vi "Download.vi"(7 "입력 클러스터":T1, 8 "에러 입력(에러 없음)":errorcluster, 10 "폴더명":path, 11 "TCP 네트워크 연결 입력":T2) -> (0 "에러 출력":errorcluster, 1 "다운로드 에러?":bool, 3 "TCP 네트워크 연결 출력":T2, 4 "타겟 경로":path, 5 "name":string, 6 "소스 경로":path)   [LabVIEW 2020]
uses:
  <vilib>/FTP/ftp0.llb/FTP Session.ctl
  <vilib>/Utility/sysdir.llb/System Directory Type.ctl
  <vilib>/security/Message Digest/API/Instances/File/SHA-256 File Checksum.vi
  <vilib>/security/Message Digest/API/NI_Message Digest API.lvlib
  <vilib>/FTP/NI_FTP.lvlib
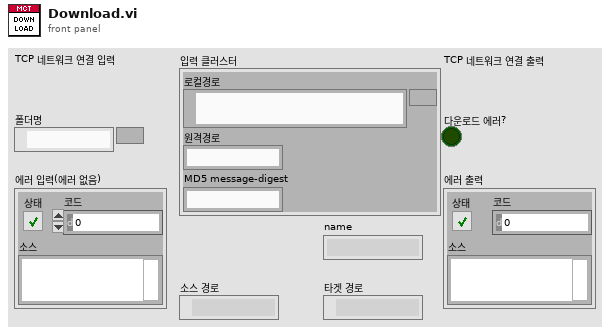
[diagram p1: front panel]
types:
  T1 = cluster{"로컬경로":path, "원격경로":string, "MD5 message-digest":string}
  T2 = typedef "NI_FTP.lvlib/FTP Session.ctl" = refnum<k5>
  T3 = typedef "System Directory Type.ctl" = i32
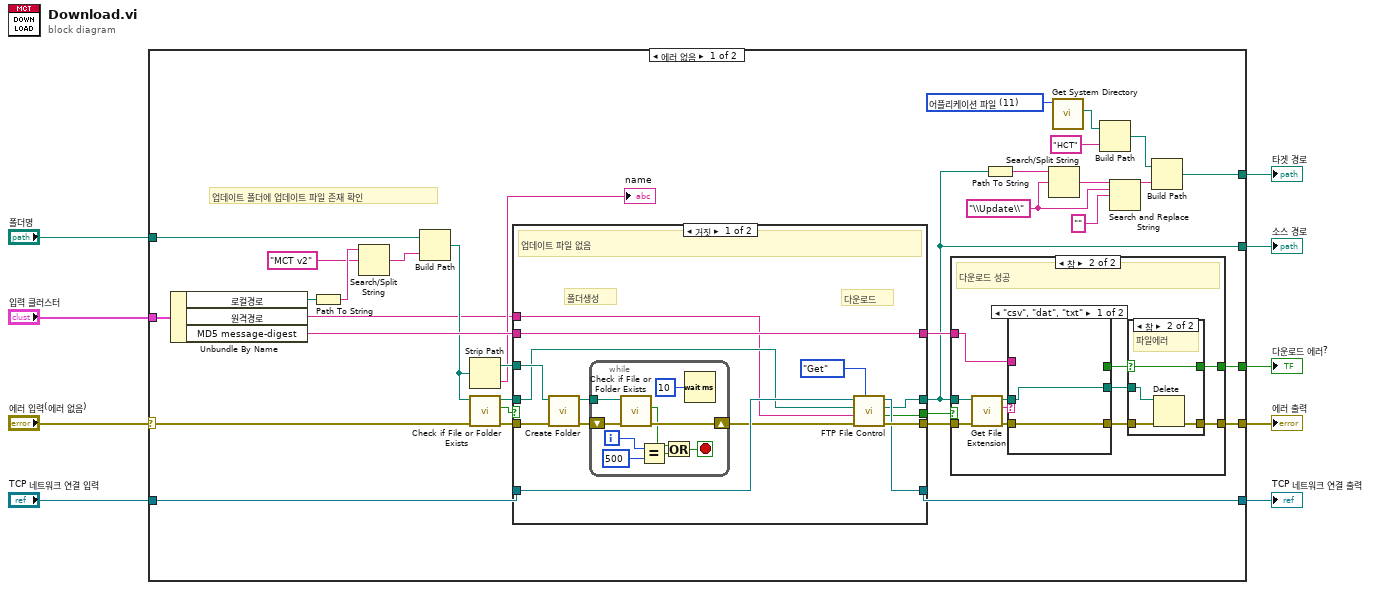
[diagram p0: block diagram]
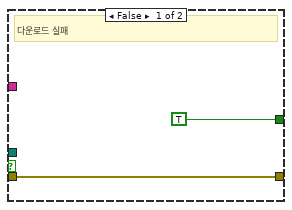
[diagram p2: hidden frame]
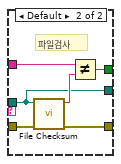
[diagram p3: hidden frame]
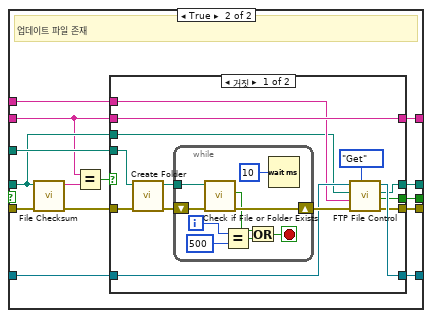
[diagram p5: hidden frame]
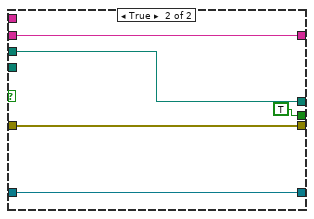
[diagram p6: hidden frame]
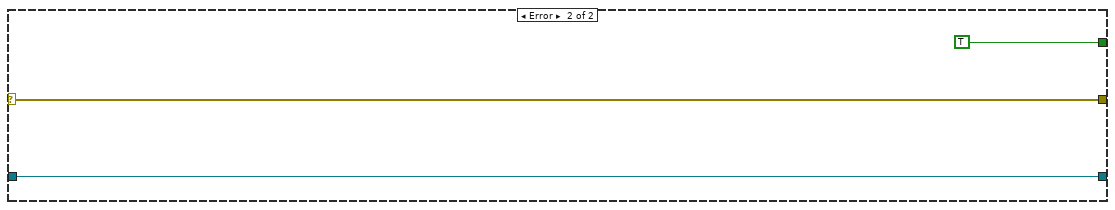
[diagram p7: hidden frame]
diagram:
  n1 = case shown="에러 없음" "에러 입력(에러 없음)" {
    selector: "에러 입력(에러 없음)" -> [w10 w135]
    tunnel: [w41 TRUE] -> w9
    tunnel: [w38 w135] -> w8
    tunnel: [w36 w137] -> w7
    tunnel: "TCP 네트워크 연결 입력" -> [w35 w137]
    tunnel: "폴더명" -> [w28 _]
    tunnel: "입력 클러스터" -> [w25 _]
    tunnel: [w21 _] -> w3
    tunnel: [w11 _] -> w2
    frame No Error {
      w16 = T3 11 items=["사용자 홈"=0, "사용자 데스크탑"=1, "사용자 문서"=2, "사용자 어플리케이션 데이터"=3, "사용자 환경"=4, "사용자 임시"=5, "퍼블릭 문서"=6, "퍼블릭 어플리케이션 데이터"=7, "퍼블릭 환경"=8, "퍼블릭 캐시"=13, "시스템 코어 라이브러리"=9, "시스템 설치된 라이브러리"=10, "어플리케이션 파일"=11, "부팅 볼륨 루트"=12] ("system directory type")
      w18 = "\\Update\\" ("검색 문자열/문자 (-)")
      # "업데이트 폴더에 업데이트 파일 존재 확인"
      n2 = Unbundle By Name(w25) -> ("로컬경로"=w24:path, "원격경로"=w23:string, "MD5 message-digest"=w40:string)
      n3 = Path To String(path=w24) -> (string=w27:string)
      n4 = Search/Split String(string=w27, search string/char (-)="MCT v2" ("검색 문자열/문자 (-)")) -> (match + rest of string=w29:string)  [unwired: 1 in, 2 out]
      n5 = Build Path(base path=w28, name or relative path=w29) -> (appended path=w39:path)
      n6 = Strip Path(path=w39) -> (stripped path=w34:path, name=→"name":string)
      n7 = call <vilib>:"Check if File or Folder Exists.vi"("error in (no error)"=w10, "path"=w39) -> ("error out"=w31:errorcluster, "file or folder exists?"=w32:bool, "dup path"=w33:path)  [unwired: 7 in]
      n8 = case shown="거짓" w32 {
        tunnel: w31 -> [w83 w106]
        tunnel: w33 -> [w71 w101]
        tunnel: w40 -> [w75 w94]
        tunnel: w34 -> [w79 w102]
        tunnel: w35 -> [w81 w100]
        tunnel: [w80 w99] -> w36
        tunnel: [w82 w98] -> w37
        tunnel: w23 -> [w70 w97]
        tunnel: [w73 w96] -> w21
        tunnel: [w74 w95] -> w42
        tunnel: [w75 w93] -> w22
        frame False {
          # "다운로드"
          # "폴더생성"
          # "업데이트 파일 없음"
          n9 = call "Create Folder.vi"("에러 입력"=w83, "폴더경로"=w79) -> ("error out"=w78:errorcluster, "dup path"=w77:path)  [unwired: 8 in]
          n10 = while {
            shift-right: [w91] -> w76
            shift-left: w78 -> [w92]
            tunnel: w77 -> [w90]
            i -> [w86]
            stop <- w88 stop-if-true
            n11 = call <vilib>:"Check if File or Folder Exists.vi"("error in (no error)"=w92, "path"=w90) -> ("error out"=w91:errorcluster, "file or folder exists?"=w89:bool)  [unwired: 7 in, 1 out]
            n12 = Equal?(x=w86, y=500) -> (x = y?=w87:bool)
            n13 = Or(x=w89, y=w87) -> (x .or. y?=w88:bool)
            n14 = Wait (ms)(milliseconds to wait=u32 10 ("대기 시간(ms)")) -> ()  [unwired: 1 out]
          }
          n15 = call "FTP File Control.vi"("Comm"=enum16{"Get", "Put"}."Get", "에러 입력"=w76, "원격경로"=w70, "로컬경로"=w71, "TCP 네트워크 연결 입력"=w81) -> ("에러 출력"=w82:errorcluster, "파일존재?"=w74:bool, "로컬경로 out"=w73:path, "TCP 네트워크 연결 출력"=w80:T2)  [unwired: 2 in, 1 out]
        }
        frame True {
          # "업데이트 파일 존재"
          n16 = call-poly <vilib>:"File Checksum.vi"("error in"=w106, "path"=w101) -> ("error out"=w103:errorcluster, "digest"=w105:string)  [unwired: 8 in]
          n17 = Equal?(x=w94, y=w105) -> (x = y?=w104:bool)
          n18 = case shown="거짓" w104 {
            tunnel: w103 -> [w120 w133]
            tunnel: w102 -> [w119 _]
            tunnel: w101 -> [w107 w132]
            tunnel: w100 -> [w115 w134]
            tunnel: [w114 w134] -> w99
            tunnel: [w113 w133] -> w98
            tunnel: w97 -> [w108 _]
            tunnel: [w110 w132] -> w96
            tunnel: [w111 TRUE ("파일존재?")] -> w95
            tunnel: w94 -> [w112 w130]
            tunnel: [w112 w130] -> w93
            frame False {
              n19 = call "Create Folder.vi"("에러 입력"=w120, "폴더경로"=w119) -> ("error out"=w118:errorcluster, "dup path"=w117:path)  [unwired: 8 in]
              n20 = while {
                shift-right: [w128] -> w116
                shift-left: w118 -> [w129]
                tunnel: w117 -> [w127]
                i -> [w123]
                stop <- w125 stop-if-true
                n21 = call <vilib>:"Check if File or Folder Exists.vi"("error in (no error)"=w129, "path"=w127) -> ("error out"=w128:errorcluster, "file or folder exists?"=w126:bool)  [unwired: 7 in, 1 out]
                n22 = Equal?(x=w123, y=500) -> (x = y?=w124:bool)
                n23 = Or(x=w126, y=w124) -> (x .or. y?=w125:bool)
                n24 = Wait (ms)(milliseconds to wait=u32 10 ("대기 시간(ms)")) -> ()  [unwired: 1 out]
              }
              n25 = call "FTP File Control.vi"("Comm"=enum16{"Get", "Put"}."Get", "에러 입력"=w116, "원격경로"=w108, "로컬경로"=w107, "TCP 네트워크 연결 입력"=w115) -> ("에러 출력"=w113:errorcluster, "파일존재?"=w111:bool, "로컬경로 out"=w110:path, "TCP 네트워크 연결 출력"=w114:T2)  [unwired: 2 in, 1 out]
            }
            frame True {
            }
          }
        }
      }
      n26 = case shown="참" w42 {
        tunnel: w37 -> [w44 w50]
        tunnel: [w44 w54] -> w38
        tunnel: w21 -> [_ w48]
        tunnel: [TRUE w52] -> w41
        tunnel: w22 -> [_ w51]
        frame False {
          # "다운로드 실패"
        }
        frame True {
          # "다운로드 성공"
          n27 = call <vilib>:"Get File Extension.vi"("error in (no error)"=w50, "file"=w48) -> ("error out"=w49:errorcluster, "lowercase file extension"=w46:string, "dup file"=w47:path)  [unwired: 5 in, 2 out]
          n28 = case shown="\"csv\", \"dat\", \"txt\"" w46 {
            tunnel: [w57 w62] -> w55
            tunnel: [_ w58] -> w53
            tunnel: w51 -> [_ w61]
            tunnel: w49 -> [w57 w60]
            tunnel: w47 -> [w56 w59]
            tunnel: [w56 w59] -> w45
            frame "csv", "dat", "txt" {
            }
            frame Default {
              # "파일검사"
              n29 = call-poly <vilib>:"File Checksum.vi"("error in"=w60, "path"=w59) -> ("error out"=w62:errorcluster, "digest"=w63:string)  [unwired: 8 in]
              n30 = Not Equal?(x=w61, y=w63) -> (x != y?=w58:bool)
            }
          }
          n31 = case shown="참" w53 {
            selector: w53 -> [w64 w67]
            tunnel: w55 -> [w65 w69]
            tunnel: w45 -> [_ w66]
            tunnel: [w65 w68] -> w54
            tunnel: [w64 w67] -> w52
            frame False {
              # "성공"
            }
            frame True {
              # "파일에러"
              n32 = Delete(path (use dialog)=w66, error in=w69) -> (error out=w68:errorcluster)  [unwired: 3 in, 2 out]
            }
          }
        }
      }
      n33 = Path To String(path=w21) -> (string=w20:string)
      n34 = Search/Split String(string=w20, search string/char (-)=w18) -> (match + rest of string=w19:string)  [unwired: 1 in, 2 out]
      n35 = call <vilib>:"Get System Directory.vi"("system directory type"=w16) -> ("system directory"=w15:path)  [unwired: 10 in]
      n36 = Build Path(base path=w15, name or relative path="HCT" ("이름 또는 상대 경로")) -> (appended path=w13:path)
      n37 = Search and Replace String(input string=w19, search string=w18, replace string="" ("대체 문자열(\"\")")) -> (result string=w12:string)  [unwired: 5 in, 3 out]
      n38 = Build Path(base path=w13, name or relative path=w12) -> (appended path=w11:path)
    }
    frame Error {
    }
  }
  "다운로드 에러?" <- w9
  "에러 출력" <- w8
  "TCP 네트워크 연결 출력" <- w7
  "타겟 경로" <- w2
  "소스 경로" <- w3
